vi "WriteRegister.vi"(8 "Divider":i32=2, 9 "WriteSize":enum16{"1", "2", "4"}(ring), 10 "RegisterValue":u32, 11 "RegisterAddress":u8) -> ()   [LabVIEW 2012]
uses:
  <vilib>/Platform/TimedLoop/XDataNode/timing_clust.ctl
  <vilib>/Platform/TimedLoop/XDataNode/nitl_modes.ctl
  <vilib>/Platform/TimedLoop/XDataNode/wakeup.ctl
  <vilib>/rvi/Emulation/niFpgaSctlEmulationRegisterWithScheduler.vi
  <vilib>/rvi/eio/common/nirviEmuTemplateMethod_errors.vi
  <vilib>/rvi/Emulation/niFpgaSctlEmulationScheduler.vi
  <vilib>/Platform/TimedLoop/XDataNode/XDataNode.xnode
  <vilib>/eio/EIONode/EIONode.xnode
  <vilib>/Platform/TimedLoop/XDataNode/XDNodeRunTimeDep.lvlib
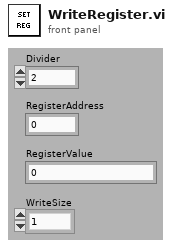
[diagram p1: front panel]
types:
  T1 = typedef "XDNodeRunTimeDep.lvlib/timing_clust.ctl" = cluster{"Expected End [f-1]":u64, "Actual End [f-1]":u64, "Finished Late? [f-1]":bool, "Expected End [i-1]":u64, "Actual End [i-1]":u64, "Finished Late? [i-1]":bool, "Expected Start [i]":u64, "Actual Start [i]":u64, "Expected Start [f]":u64, "Actual Start [f]":u64, "Source Name":string, "Structure Name":string, "Period":i64, "Deadline":i64, "Offset":i64, "Start":i64, "Priority":i32, "Timeout":i32, "Mode":T2, "Wakeup Reason":T3, "Error":errorcluster, "Source Type":string, "Secondary Source Type":string, "Global End Time":u64, "Global Start Time":u64, "Frame Duration":u64, "Iteration Duration":u64, "Assigned CPU":i32, "I/O Scan Engine Mode":u32}
  T2 = typedef "XDNodeRunTimeDep.lvlib/nitl_modes.ctl" = enum32{"No Change", "Process missed periods, maintain original phase", "Discard missed periods, maintain original phase", "Process missed periods, ignore original phase", "Discard missed periods, ignore original phase"}
  T3 = typedef "XDNodeRunTimeDep.lvlib/wakeup.ctl" = enum32{"Normal", "Aborted", "Asynchronous wakeup", "Timing source error", "Timed loop error", "Timeout"}
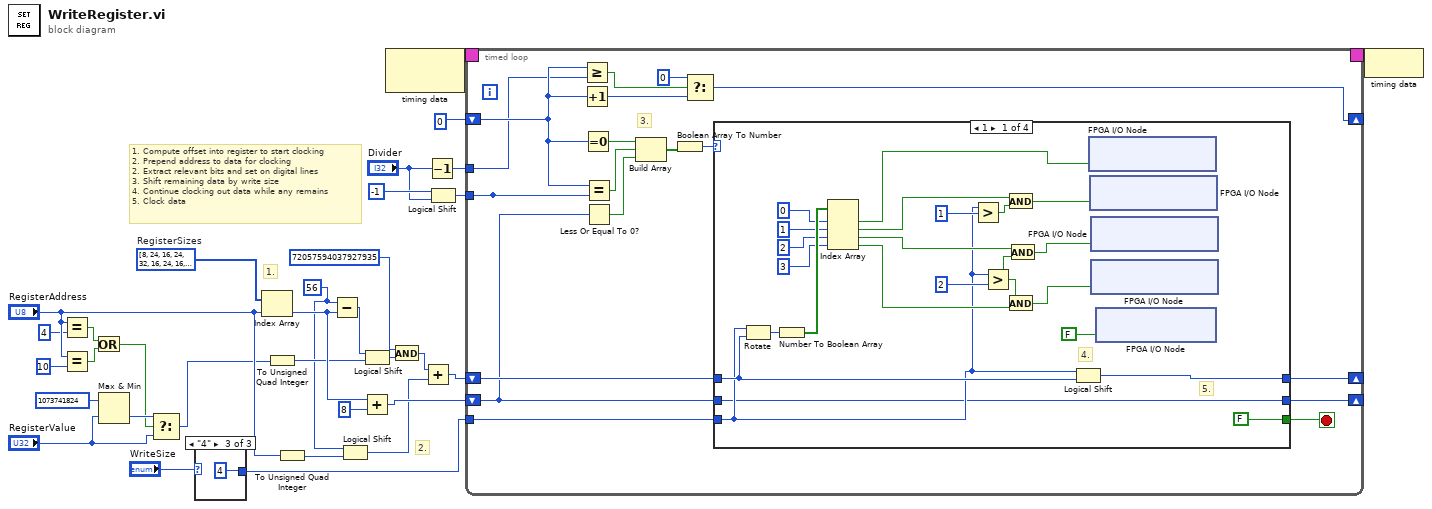
[diagram p0: block diagram]
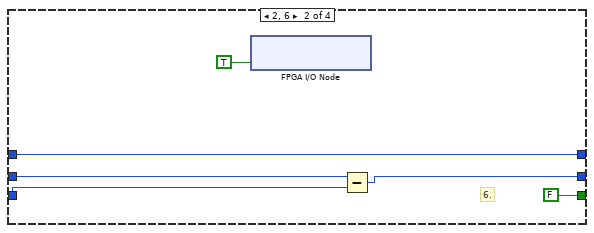
[diagram p2: hidden frame]
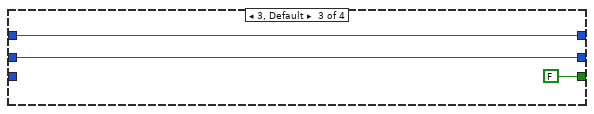
[diagram p3: hidden frame]
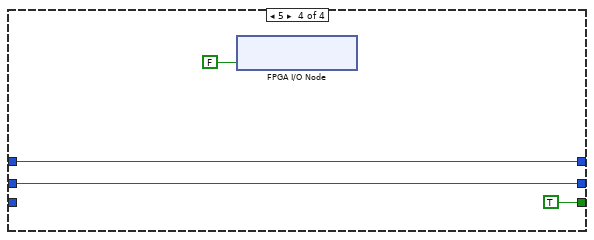
[diagram p4: hidden frame]
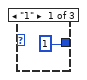
[diagram p5: hidden frame]
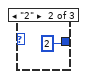
[diagram p6: hidden frame]
diagram:
  w23 = 56 ("x")
  w32 = i16[] [8, 24, 16, 24, 32, 16, 24, 16, 32, 32, 32, 32, 32, 32, 32, 32, 32, 32, 32, 32, 32, 32, 32, 32, 32]  # RegisterSizes
  # "2."
  # "1. Compute offset into register to start clocking\n2. Prepend address to data for clocking\n2. Extract relevant bits and set on digital lines\n3. Shift remaining data by write size\n4. Continue clocking out data while any remains\n5. Clock data"
  # "1."
  n1 = Equal?(x="RegisterAddress", y=u8 4) -> (x = y?=w7:bool)
  n2 = Equal?(x="RegisterAddress", y=u8 10) -> (x = y?=w6:bool)
  n3 = Or(x=w7, y=w6) -> (x .or. y?=w2:bool)
  n4 = Max & Min(x=u32 1073741824, y="RegisterValue") -> (min(x,y)=w4:u32)  [unwired: 1 out]
  n5 = Select(t=w4, s=w2, f="RegisterValue") -> (s? t:f=w1:u32)
  n6 = case shown="\"4\"" "WriteSize" {
    tunnel: [i16 1 i16 2 i16 4] -> w29
    frame "1" {
    }
    frame "2" {
    }
    frame "4" {
    }
  }
  n7 = Index Array(array=w32, index="RegisterAddress") -> (element=w28:i16)
  n8 = To Unsigned Quad Integer(1:w1) -> (0:w25:u64)
  n9 = To Unsigned Quad Integer(1:"RegisterAddress") -> (0:w19:u64)
  n10 = Subtract(x=w23, y=w28) -> (x-y=w31:i32)
  n11 = Logical Shift(y=w23, x=w19) -> (x << y=w18:u64)
  n12 = Logical Shift(y=w31, x=w25) -> (x << y=w22:u64)
  n13 = Add(x=w28, y=i16 8) -> (x+y=w27:i16)
  n14 = node-c288() -> (w17:T1)  [unwired: 1 in]
  n15 = And(x=u64 72057594037927935, y=w22) -> (x .and. y?=w21:u64)
  n16 = Add(x=w21, y=w18) -> (x+y=w24:u64)
  n17 = Decrement(x="Divider") -> (x-1=w11:i32)
  n18 = Logical Shift(y=i8 -1, x="Divider") -> (x << y=w14:i32)
  n19 = timed-loop {
    shift-right: [w51] -> _
    shift-left: w24 -> [w50]
    tunnel: w29 -> [w38]
    shift-right: [w52] -> _
    shift-left: w27 -> [w37]
    timing: w17 -> [_]
    timing-out: [_] -> w16
    tunnel: w11 -> [w43]
    tunnel: [w49] -> _
    tunnel: w14 -> [w49]
    shift-right: [w39] -> _
    shift-left: i16 0 -> [w44]
    stop <- w53 stop-if-true
    # "3."
    n20 = Greater Or Equal?(x=w44, y=w43) -> (x >= y?=w42:bool)
    n21 = Increment(x=w44) -> (x+1=w41:i16)
    n22 = Equal To 0?(x=w44) -> (x = 0?=w48:bool)
    n23 = Equal?(x=w44, y=w49) -> (x = y?=w47:bool)
    n24 = Less Or Equal To 0?(x=w37) -> (x <= 0?=w36:bool)
    n25 = Build Array(w48, w47, w36) -> (w46:bool[])
    n26 = Boolean Array To Number(Boolean array=w46) -> (number=w45:u8)
    n27 = Select(t=i16 0, s=w42, f=w41) -> (s? t:f=w39:i16)
    n28 = case shown="1" w45 {
      tunnel: w37 -> [w54 w79 w85 w86]
      tunnel: [FALSE FALSE FALSE TRUE] -> w53
      tunnel: [w54 w77 w85 w86] -> w52
      tunnel: [w76 w81 w84 w87] -> w51
      tunnel: w50 -> [w69 w81 w84 w87]
      tunnel: w38 -> [w57 w78 _ _]
      frame 1 {
        # "5."
        # "4."
        n29 = Rotate(1:w69, 2:w57) -> (0:w71:u64)
        n30 = Number To Boolean Array(number=w71) -> (Boolean array=w70:bool[])
        n31 = Index Array(array=w70, index #1=0 ("index"), index #2=1 ("index"), index #3=2 ("index"), index #4=3 ("index")) -> (element #1=w65:bool, element #2=w68:bool, element #3=w67:bool, element #4=w66:bool)
        n32 = Greater?(x=w57, y=i16 1) -> (0:w75:bool)
        n33 = Greater?(x=w57, y=i16 2) -> (0:w73:bool)
        n34 = And(x=w68, y=w75) -> (x .and. y?=w64:bool)
        n35 = And(x=w73, y=w66) -> (x .and. y?=w62:bool)
        n36 = And(x=w67, y=w73) -> (x .and. y?=w63:bool)
        n37 = Logical Shift(y=w57, x=w69) -> (x << y=w76:u64)
        n38 = xnode "FPGA I/O Node"("IO Module\\SDIO0"=w65) -> ()  [unwired: 1 in, 1 out]
        n39 = xnode "FPGA I/O Node"("IO Module\\SDIO1"=w64) -> ()  [unwired: 1 in, 1 out]
        n40 = xnode "FPGA I/O Node"("IO Module\\SDIO2"=w63) -> ()  [unwired: 1 in, 1 out]
        n41 = xnode "FPGA I/O Node"("IO Module\\SDIO3"=w62) -> ()  [unwired: 1 in, 1 out]
        n42 = xnode "FPGA I/O Node"("IO Module\\SCLK"=FALSE ("IO Module\\DDCA_DIO4_Write")) -> ()  [unwired: 1 in, 1 out]
      }
      frame 2, 6 {
        # "6."
        n43 = xnode "FPGA I/O Node"("IO Module\\SCLK"=TRUE ("IO Module\\DDCA_DIO4_Write")) -> ()  [unwired: 1 in, 1 out]
        n44 = Subtract(x=w79, y=w78) -> (x-y=w77:i16)
      }
      frame 3, Default {
      }
      frame 5 {
        n45 = xnode "FPGA I/O Node"("IO Module\\SCLK"=FALSE ("IO Module\\DDCA_DIO4_Write")) -> ()  [unwired: 1 in, 1 out]
      }
    }
  }
  n46 = node-c288(w16) -> ()
